vi "chainCommands.vi"(9 "Command":string, 10 "Comments":string, 11 "StringIn":string) -> (3 "StringOut":string)   [LabVIEW 2013]
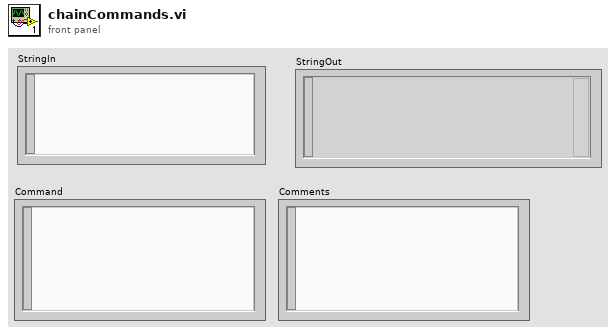
[diagram p1: front panel]
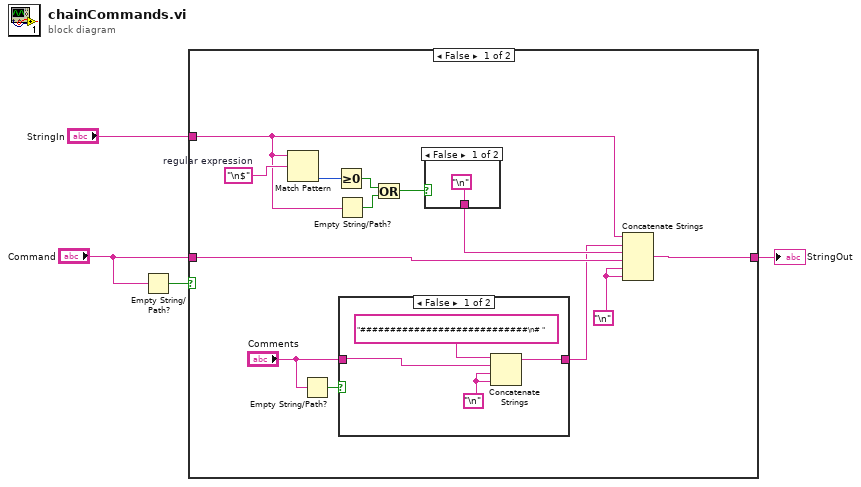
[diagram p0: block diagram]
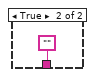
[diagram p3: hidden frame]
diagram:
  n1 = Empty String/Path?(string/path="Command") -> (empty?=w1:bool)
  n2 = case shown="False" w1 {
    tunnel: [w17 w25] -> w4
    tunnel: "StringIn" -> [w12 w25]
    tunnel: "Command" -> [w9 _]
    frame False {
      w16 = "\n$"  # regular expression
      w8 = "\n"
      n3 = Match Pattern(string=w12, regular expression=w16) -> (offset past match=w15:i32)  [unwired: 1 in, 3 out]
      n4 = Empty String/Path?(string/path="Comments") -> (empty?=w7:bool)
      n5 = Greater Or Equal To 0?(x=w15) -> (x >= 0?=w13:bool)
      n6 = Empty String/Path?(string/path=w12) -> (empty?=w10:bool)
      n7 = case shown="False" w7 {
        tunnel: [w21 w22] -> w6
        tunnel: "Comments" -> [w19 w22]
        frame False {
          w18 = "\n"
          n8 = Concatenate Strings("############################\n# ", w19, w18, w18) -> (w21:string)
        }
        frame True {
        }
      }
      n9 = Or(x=w13, y=w10) -> (x .or. y?=w11:bool)
      n10 = case shown="False" w11 {
        tunnel: ["\n" ""] -> w14
        frame False {
        }
        frame True {
        }
      }
      n11 = Concatenate Strings(w12, w6, w14, w9, w8, w8) -> (w17:string)
    }
    frame True {
    }
  }
  "StringOut" <- w4
